vi "Export_mappingFileName v10.5.1.vi"(0 "ITC503 Current Values":T3 {"ITC503 Gradient" format="%.2f"; "ITC503 Setpoint" min=-273.0 max=300000.0 step=0.0001 format="%.1f"; "ITC503 I" format="%_1f"; "ITC503 P" format="%_1f"; "ITC503 Temperature" min=0.0 max=1645.0 step=1e-05 format="%.2f"; "ITC503 Heater" min=0.0 max=100.0 step=0.01 scale=0.0..100.0}, 1 "iHR Current Values":T4={"iHR 550 Front Entrance"=0.0, "iHR550 Side Exit"=0.0, "iHR550 Wavelength"=897.9988, "iHR550 Exit Mirror"=2, "iHR550 Grating"="1", "Grating Index"=1} {"iHR550 Exit Mirror" items=["EntranceMirror", "ExitMirror", "Front", "Side"]}, 2 "Spectra Settings":T2={"Integration Time"=10.0, "Repetitions"=10, "Mapping Spectra"=TRUE} caption="Mapping Spectra Settings" {"Repetitions" min=1 max=100 step=1; "Integration Time" min=0.5 max=6000.0 step=1.0 format="%.1f"}, 3 "Mapping Parameters":T1={"X Start Position"=0.0, "X Stop Position"=10.0, "Y Start Position"=0.0, "Y Stop Position"=10.0, "Step Size"=1.0} {"Step Size" min=0.1 max=30.0 step=0.1 format="%.1f"; "Y Stop Position" min=0.0 max=30.0 step=0.1 format="%.1f"; "Y Start Position" min=0.0 max=30.0 step=0.1 format="%.1f"; "X Stop Position" min=0.0 max=30.0 step=0.1 format="%.1f"; "X Start Position" min=0.0 max=30.0 step=0.1 format="%.1f"}) -> (5 "Filename":string)   [LabVIEW 2010]
uses:
  iHR550/TypeDefs/iHR Current Values.ctl
  ITC503/TypeDefs/ITC503 Current Values.ctl
  Mapping/TypeDefs/Mapping Spectra Params.ctl
  Mapping/TypeDefs/Mapping Drive Params.ctl
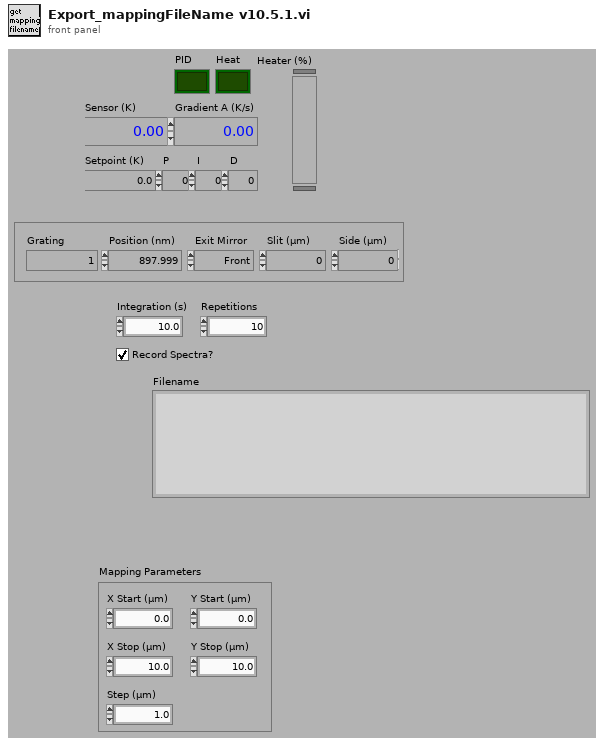
[diagram p1: front panel]
types:
  T1 = typedef "Mapping Drive Params.ctl" = cluster{"X Start Position":dbl, "X Stop Position":dbl, "Y Start Position":dbl, "Y Stop Position":dbl, "Step Size":dbl}
  T2 = typedef "Mapping Spectra Params.ctl" = cluster{"Integration Time":dbl, "Repetitions":u16, "Mapping Spectra":bool}
  T3 = typedef "ITC503 Current Values.ctl" = cluster{"ITC503 Heater":dbl, "ITC503 Temperature":dbl, "ITC503 P":dbl, "ITC503 I":dbl, "ITC503 D":dbl, "ITC503 Setpoint":dbl, "ITC503 Gradient":dbl, "ITC503 Heater Auto":bool, "ITC503 PID Auto":bool}
  T4 = typedef "iHR Current Values.ctl" = cluster{"iHR 550 Front Entrance":dbl, "iHR550 Side Exit":dbl, "iHR550 Wavelength":dbl, "iHR550 Exit Mirror":i32, "iHR550 Grating":string, "Grating Index":i32}
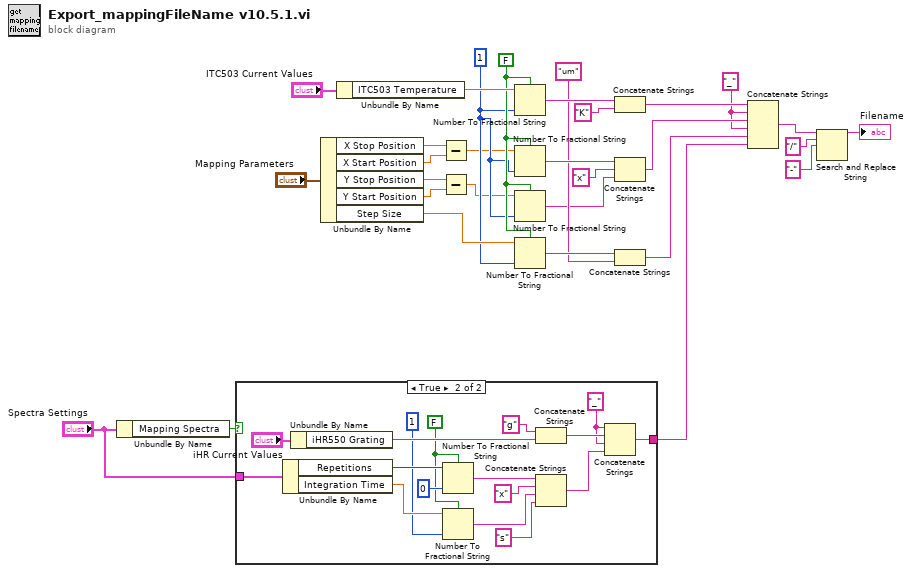
[diagram p0: block diagram]
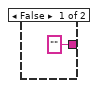
[diagram p2: hidden frame]
diagram:
  w10 = "_" ("String")
  w19 = FALSE ("Systemdezimalzeichen verwenden (T)")
  w5 = i16 1 ("Genauigkeit (6)")
  n1 = Unbundle By Name("Spectra Settings") -> ("Mapping Spectra"=w20:bool)
  n2 = case shown="True" w20 {
    tunnel: "Spectra Settings" -> [_ w38]
    tunnel: ["" w35] -> w12
    frame False {
    }
    frame True {
      w34 = "_" ("String")
      w33 = FALSE ("use system decimal point (T)")
      n3 = Unbundle By Name(w38) -> ("Repetitions"=w47:u16, "Integration Time"=w42:dbl)
      n4 = Unbundle By Name("iHR Current Values") -> ("iHR550 Grating"=w40:string)
      n5 = Number To Fractional String(use system decimal point (T)=w33, number=w47, precision (6)=i16 0 ("Genauigkeit (6)")) -> (F-format string=w45:string)  [unwired: 1 in]
      n6 = Number To Fractional String(use system decimal point (T)=w33, number=w42, precision (6)=i16 1) -> (F-format string=w44:string)  [unwired: 1 in]
      n7 = Concatenate Strings("g" ("String"), w40) -> (w36:string)
      n8 = Concatenate Strings(w45, "x" ("String"), w44, "s" ("String")) -> (w32:string)
      n9 = Concatenate Strings(w34, w36, w34, w32) -> (w35:string)
    }
  }
  n10 = Unbundle By Name("Mapping Parameters") -> ("X Stop Position"=w9:dbl, "X Start Position"=w8:dbl, "Y Stop Position"=w7:dbl, "Y Start Position"=w6:dbl, "Step Size"=w18:dbl)
  n11 = Unbundle By Name("ITC503 Current Values") -> ("ITC503 Temperature"=w29:dbl)
  n12 = Subtract(x=w9, y=w8) -> (x-y=w4:dbl)
  n13 = Subtract(x=w7, y=w6) -> (x-y=w3:dbl)
  n14 = Number To Fractional String(use system decimal point (T)=w19, number=w29, precision (6)=w5) -> (F-format string=w28:string)  [unwired: 1 in]
  n15 = Number To Fractional String(use system decimal point (T)=w19, number=w4, precision (6)=w5) -> (F-format string=w26:string)  [unwired: 1 in]
  n16 = Number To Fractional String(use system decimal point (T)=w19, number=w3, precision (6)=w5) -> (F-format string=w2:string)  [unwired: 1 in]
  n17 = Number To Fractional String(use system decimal point (T)=w19, number=w18, precision (6)=w5) -> (F-format string=w17:string)  [unwired: 1 in]
  n18 = Concatenate Strings(w28, "K" ("String")) -> (w15:string)
  n19 = Concatenate Strings(w26, "x" ("string"), w2) -> (w14:string)
  n20 = Concatenate Strings(w17, "um" ("String")) -> (w13:string)
  n21 = Concatenate Strings(w15, w10, w14, w10, w13, w12) -> (w25:string)
  n22 = Search and Replace String(input string=w25, search string="/" ("Such-String"), replace string="-" ("replace string (\"\")")) -> (result string=→"Filename":string)  [unwired: 5 in, 3 out]
